vi "Test Variant to Objects.vi"() -> ()   [LabVIEW 2021]
uses:
  <vilib>/TSA/Abstract Data Classes/Abs_Types/Value/Abs_Value.lvclass
  C:/Program Files (x86)/National Instruments/LabVIEW 2021/vi.lib/TSA/Abstract Data Classes/Abs_Types/Type/Abs_Type.lvclass
  <vilib>/TSA/Abstract Data Classes/Abs_Types/Time/Support/Type.ctl
  <vilib>/TSA/Abstract Data Classes/Abs_Types/Waveform/Abs_Waveform.lvclass
  <vilib>/TSA/Abstract Data Classes/Abs_Types/Boolean/Abs_Boolean.lvclass
  <vilib>/TSA/Abstract Data Classes/Abs_Types/I32 Integer/Abs_I32 Integer.lvclass
  <vilib>/TSA/Abstract Data Classes/Abs_Types/String/Abs_String.lvclass
  <vilib>/TSA/Omni-Bus/Local Bus/Support/Tag List Type.ctl
  <vilib>/Utility/Data Type/Type Definitions/Data Type.ctl
  <vilib>/TSA/Omni-Bus/Local Bus/Local Bus.lvclass
  C:/Program Files (x86)/National Instruments/LabVIEW 2021/vi.lib/TSA/Omni-Bus/Omni-Bus/Bus Access/Bus_Access.lvclass
  <vilib>/TSA/Omni-Bus/Omni-Bus/Omni_Bus.lvclass
  <vilib>/TSA/Abstract Data Classes/Abs_Types/Double Float/Abs_Double Float.lvclass
  <vilib>/TSA/Abstract Data Classes/Abs_Types/Time/Abs_Time.lvclass
  <vilib>/TSA/Abstract Data Classes/Abs_Types/Type/Abs_Type.lvclass/Abs_Type.ctl
  <vilib>/TSA/Omni-Bus/Omni-Bus/Omni_Bus.lvclass/Omni_Bus.ctl
  <vilib>/TSA/Omni-Bus/Omni-Bus/Support/Get/Get DBL.vi
  <vilib>/TSA/Omni-Bus/Omni-Bus/Support/Write/Write DBL.vi
  <vilib>/TSA/Abstract Data Classes/Abs_Types/Time/Simple Read.vi
  <vilib>/TSA/Abstract Data Classes/Abs_Types/Double Float/Simple Read.vi
  <vilib>/TSA/Abstract Data Classes/Abs_Types/String/Simple Read.vi
  <vilib>/TSA/Abstract Data Classes/Abs_Types/I32 Integer/Simple Read.vi
  <vilib>/TSA/Abstract Data Classes/Abs_Types/Boolean/Simple Read.vi
  <vilib>/TSA/Abstract Data Classes/Abs_Types/Waveform/Simple Read.vi
  <vilib>/TSA/Omni-Bus/Omni-Bus/Support/FindVar.vi
  <vilib>/Utility/error.llb/Clear Errors.vi
  <vilib>/TSA/Omni-Bus/Omni-Bus/Properties/Read Var Map.vi
  <vilib>/TSA/Abstract Data Classes/Abs_Types/Type/Properties/Read Tag.vi
  <vilib>/TSA/Omni-Bus/Omni-Bus/Support/Check For Read Only Error.vi
  <vilib>/TSA/Omni-Bus/Omni-Bus/Support/Incorrect Tag String Error.vi
  <vilib>/Utility/error.llb/Error Cluster From Error Code.vi
  <vilib>/TSA/Abstract Data Classes/Abs_Types/Type/Abs_Type.lvclass
  <vilib>/ErrorRing/Error Ring.xnode
  Source/Support/Nodes/Leaves/Synch/With Values/WaitOn/bt_WaitOn_Synch_WithValues.lvclass
  <vilib>/measure/NI_MABase.lvlib
  <vilib>/Utility/Data Type/NI_Data Type.lvlib
  C:/Program Files (x86)/National Instruments/LabVIEW 2021/vi.lib/TSA/Omni-Bus/Local Bus/Local Bus.lvclass
panel:
  out "Value 3":T1
  out "current time":timestamp
  in  "Numeric":dbl
  in  "stop":bool
  out "Value 2":dbl
  out "String":string
  out "Value":i32
  out "Boolean":bool
  out "Waveform Graph":waveform(dbl)(graph)
  out "Names OUT":string[](array[string])
  out "Value Objects OUT":refnum<class "Abs_Value.lvclass">[](array[class])
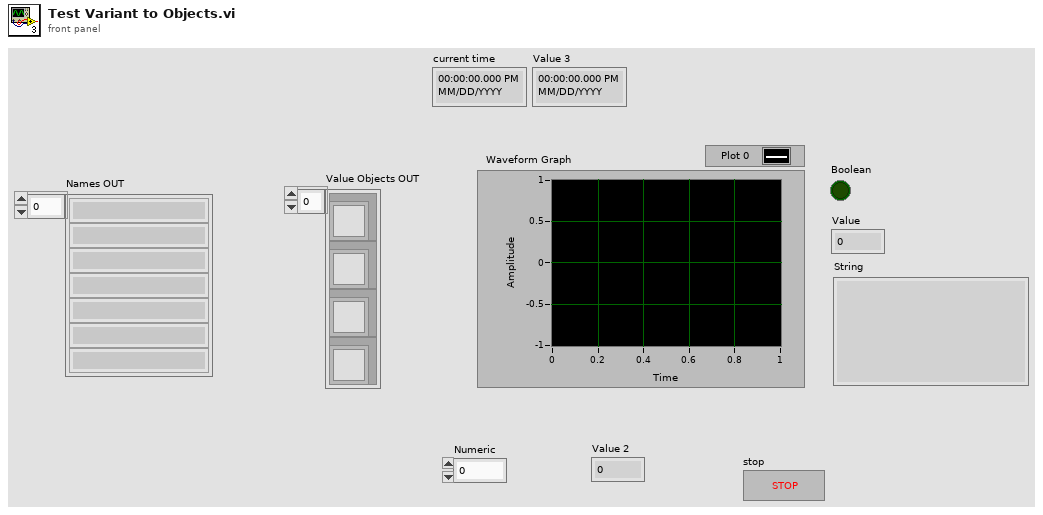
[diagram p1: front panel]
types:
  T1 = typedef "Abs_Time.lvclass/Type.ctl" = timestamp
  T2 = typedef "Local Bus.lvclass/Tag List Type.ctl" = cluster{"Tag":string, "Type":T3}
  T3 = typedef "NI_Data Type.lvlib/Data Type.ctl" = enum8{"Invalid Type", "Void", "I8", "I16", "I32", "I64", "U8", "U16", "U32", "U64", "Single Float", "Double Float", "Extended Float", "Single Complex", "Double Complex", "Extended Complex", "Enum U8", "Enum U16", "Enum U32", "Enum U64", "Single Float With Unit", "Double Float With Unit", "Extended Float With Unit", "Single Complex with Unit", "Double Complex with Unit", "Extended Complex with Unit", "Boolean", "String", "Path", "Picture", "Tag", "Array", "Cluster", "Variant", "LV Variant", "Waveform", "Timestamp", "Digital Waveform", "Digital Data", "ExpressData", "Refnum", "External Data", "VI", "Poly VI", "LabVIEW Class Instance", "Fixed Point", "Set Collection", "Map Collection"}
  T4 = cluster{"signal out":waveform(dbl), "error out":errorcluster, "Value Out":refnum<class "Abs_Double Float.lvclass">, "seconds since 1Jan1904":timestamp}
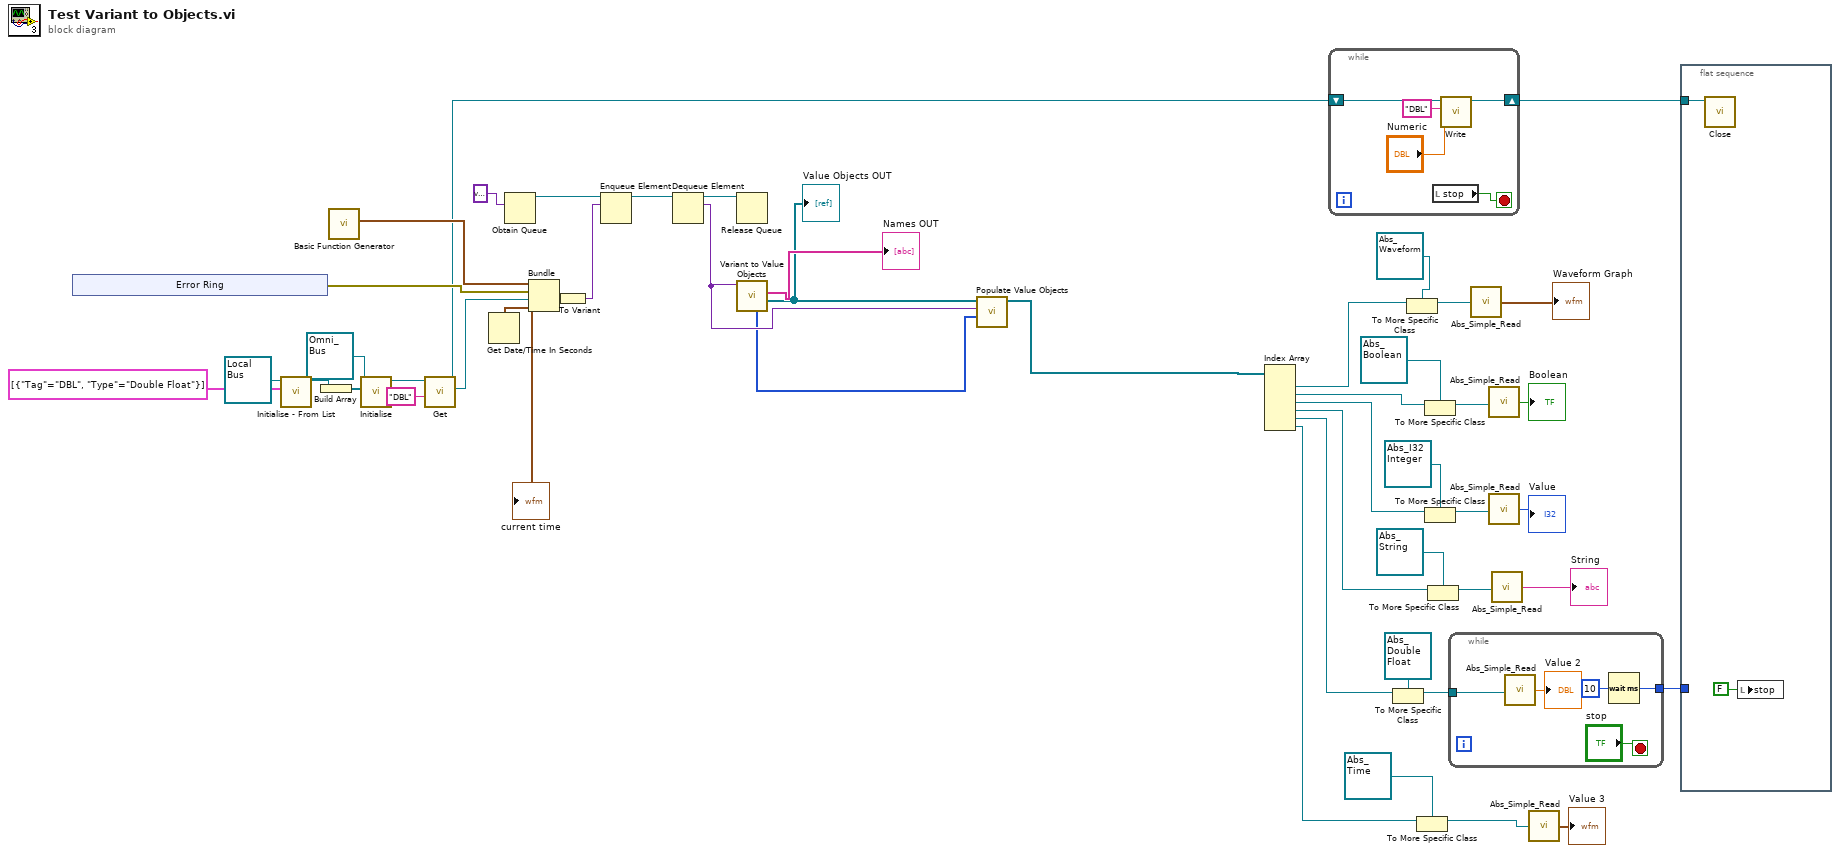
[diagram p0: block diagram]
diagram:
  n1 = xnode "Error Ring"() -> ("error out"=w47:errorcluster)
  n2 = call <vilib>:"Initialise - From List.vi"("Tag List"=T2[] [{"Tag"="DBL", "Type"=enum."Double Float"}], "Local Bus in"=refnum<class "Local Bus.lvclass"> refnum) -> ("Local Bus out"=w27:refnum<class "Local Bus.lvclass">)  [unwired: 8 in, 1 out]
  n3 = Build Array(w27) -> (w26:refnum<class "Local Bus.lvclass">[])
  n4 = call <vilib>:"Basic Function Generator.vi"() -> ("signal out"=w46:waveform(dbl))  [unwired: 9 in, 2 out]
  n5 = call-dynamic "Initialise.vi"("Bus Access"=w26, "Var Bus in"=refnum<class "Omni_Bus.lvclass"> refnum) -> ("Var Bus out"=w24:refnum<class "Omni_Bus.lvclass">)  [unwired: 8 in, 1 out]
  n6 = call-poly <vilib>:"Get.vi"("Tag"="DBL", "Var Bus in"=w24) -> ("Value Out"=w22:refnum<class "Abs_Double Float.lvclass">, "Var Bus out"=w18:refnum<class "Omni_Bus.lvclass">)  [unwired: 6 in, 2 out]
  n7 = Get Date/Time In Seconds() -> (seconds since 1Jan1904=w15:timestamp)
  "current time" <- w15
  n8 = Obtain Queue(element data type=variant) -> (queue out=w9:refnum<queue>)  [unwired: 4 in, 2 out]
  n9 = Bundle("signal out"=w46, "error out"=w47, "Value Out"=w22, "seconds since 1Jan1904"=w15) -> (w48:T4)  [unwired: 1 in]
  n10 = To Variant(anything=w48) -> (Variant=w8:variant)
  n11 = Enqueue Element(queue=w9, element=w8) -> (queue out=w5:refnum<queue>)  [unwired: 2 in, 2 out]
  n12 = Dequeue Element(queue=w5) -> (queue out=w7:refnum<queue>, element=w3:variant)  [unwired: 2 in, 2 out]
  n13 = Release Queue(queue=w7) -> ()  [unwired: 2 in, 3 out]
  n14 = call "Variant to Value Objects.vi"("Variant"=w3) -> ("Value Objects OUT"=w4:refnum<class "Abs_Value.lvclass">[], "Names OUT"=→"Names OUT":string[], "types out"=w2:T3[])  [unwired: 7 in, 1 out]
  "Value Objects OUT" <- w4
  n15 = call "Populate Value Objects.vi"("LabVIEW types"=w2, "Variant"=w3, "Value Objects Type"=w4) -> ("Value Objects Out"=w1:refnum<class "Abs_Value.lvclass">[])  [unwired: 7 in, 1 out]
  n16 = Index Array(array=w1) -> (element #1=w45:refnum<class "Abs_Value.lvclass">, element #2=w41:refnum<class "Abs_Value.lvclass">, element #3=w36:refnum<class "Abs_Value.lvclass">, element #4=w34:refnum<class "Abs_Value.lvclass">, element #5=w19:refnum<class "Abs_Value.lvclass">, element #6=w14:refnum<class "Abs_Value.lvclass">)  [unwired: 6 in]
  n17 = while {
    shift-right: [w52] -> w16
    shift-left: w18 -> [w53]
    stop <- w49 stop-if-true
    n18 = local read "stop"() -> (w49:bool)
    n19 = call-poly <vilib>:"Write.vi"("Numeric"="Numeric", "Tag"="DBL", "Omni_Bus in"=w53) -> ("Omni_Bus out"=w52:refnum<class "Omni_Bus.lvclass">)  [unwired: 7 in, 1 out]
  }
  n20 = To More Specific Class(target class=refnum<class "Abs_Double Float.lvclass"> refnum ("Class"), reference=w19) -> (specific class reference=w20:refnum<class "Abs_Double Float.lvclass">)  [unwired: 1 in, 1 out]
  n21 = To More Specific Class(target class=refnum<class "Abs_Waveform.lvclass"> refnum ("Abs_Waveform in"), reference=w45) -> (specific class reference=w43:refnum<class "Abs_Waveform.lvclass">)  [unwired: 1 in, 1 out]
  n22 = To More Specific Class(target class=refnum<class "Abs_Time.lvclass"> refnum ("Class"), reference=w14) -> (specific class reference=w12:refnum<class "Abs_Time.lvclass">)  [unwired: 1 in, 1 out]
  n23 = To More Specific Class(target class=refnum<class "Abs_Boolean.lvclass"> refnum ("Boolean in"), reference=w41) -> (specific class reference=w40:refnum<class "Abs_Boolean.lvclass">)  [unwired: 1 in, 1 out]
  n24 = To More Specific Class(target class=refnum<class "Abs_I32 Integer.lvclass"> refnum ("Class"), reference=w36) -> (specific class reference=w37:refnum<class "Abs_I32 Integer.lvclass">)  [unwired: 1 in, 1 out]
  n25 = To More Specific Class(target class=refnum<class "Abs_String.lvclass"> refnum ("Abs_String in"), reference=w34) -> (specific class reference=w35:refnum<class "Abs_String.lvclass">)  [unwired: 1 in, 1 out]
  n26 = while {
    tunnel: w20 -> [w55]
    tunnel: [w54] -> w17
    stop <- "stop" stop-if-true
    n27 = call-poly <vilib>:"Abs_Simple_Read.vi"("Class"=w55) -> ("Value"=→"Value 2":dbl)  [unwired: 4 in]
    n28 = Wait (ms)(milliseconds to wait=u32 10) -> (millisecond timer value=w54:u32)
  }
  n29 = call-poly <vilib>:"Abs_Simple_Read.vi"("Abs_Waveform in"=w43) -> ("Waveform"=→"Waveform Graph":waveform(dbl))  [unwired: 4 in]
  n30 = call-poly <vilib>:"Abs_Simple_Read.vi"("Boolean in"=w40) -> ("Boolean"=→"Boolean":bool)  [unwired: 4 in]
  n31 = call-poly <vilib>:"Abs_Simple_Read.vi"("Class"=w37) -> ("Value"=→"Value":i32)  [unwired: 4 in]
  n32 = call-poly <vilib>:"Abs_Simple_Read.vi"("Abs_String in"=w35) -> ("String"=→"String":string)  [unwired: 4 in]
  n33 = call-poly <vilib>:"Abs_Simple_Read.vi"("Class"=w12) -> ("Value"=→"Value 3":T1)  [unwired: 4 in]
  n34 = flat-sequence {
    tunnel: w17 -> [_]
    tunnel: w16 -> [w60]
    frame #0 {
      n35 = call-dynamic "Close.vi"("Data in"=w60) -> ()  [unwired: 9 in, 2 out]
      n36 = local write "stop"(FALSE ("stop")) -> ()
    }
  }
